vi "Get Library Version.vi"(8 "error in (no error)":errorcluster, 11 "Potentiostat Galvanostat in":refnum<class "Potentiostat Galvanostat.lvclass">) -> (0 "error out":errorcluster, 2 "Version":string, 3 "Potentiostat Galvanostat out":refnum<class "Potentiostat Galvanostat.lvclass">)   [LabVIEW 2018, in "Potentiostat Galvanostat.lvclass"]
uses:
  Potentiostat Galvanostat.lvclass
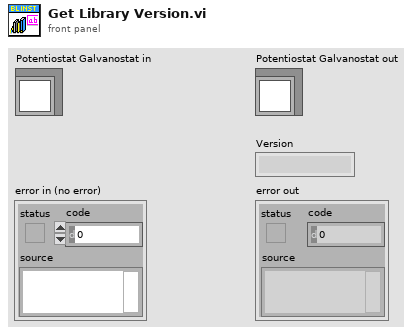
[diagram p1: front panel]
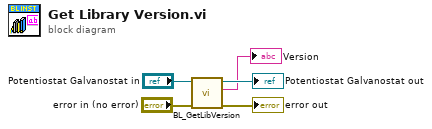
[diagram p0: block diagram]
diagram:
  n1 = call "BL_GetLibVersion.vi"("error in (no error)"="error in (no error)", "Potentiostat Galvanostat in"="Potentiostat Galvanostat in") -> ("error out"=→"error out":errorcluster, "Version"=→"Version":string, "Potentiostat Galvanostat out"=→"Potentiostat Galvanostat out":refnum<class "Potentiostat Galvanostat.lvclass">)  [unwired: 7 in]
